vi "Untitled 1.vi"() -> ()   [LabVIEW 2018]
uses:
  <vilib>/userdefined/High Color/IMAQdx.ctl
  <vilib>/vision/driver/NI_Vision_Acquisition_Software.lvlib
  <resource>/objmgr/imaqdx.rc
  <vilib>/vision/NI_Vision_Development_Module.lvlib
panel:
  in  "Blue or Luma or Val or Inten Range":cluster{"Lower value":i32, "Upper value":i32}={"Lower value"=0, "Upper value"=255}
  in  "Green or Sat Range":cluster{"Lower value":i32, "Upper value":i32}={"Lower value"=0, "Upper value"=255}
  in  "Red or Hue Range":cluster{"Lower value":i32, "Upper value":i32}={"Lower value"=0, "Upper value"=255}
  in  "Stop (F)":bool
  out "Image Out":T1(plugin-control)
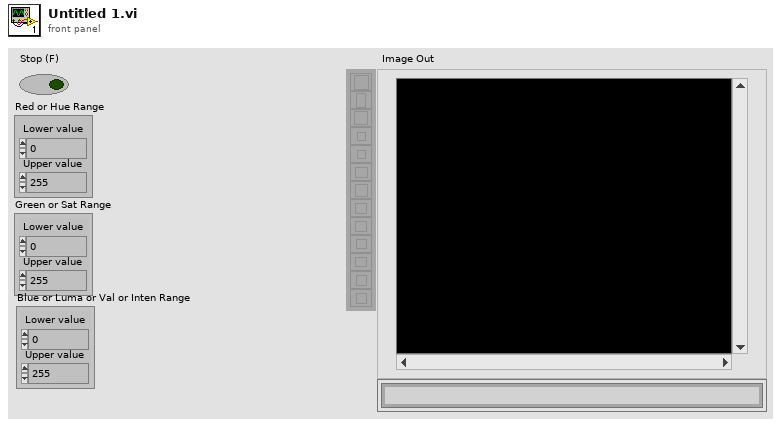
[diagram p1: front panel]
types:
  T1 = typedef "IMAQ Image.ctl" = refnum<image>
  T2 = typedef "IMAQdx.ctl" = refnum<k21>
  T3 = typedef "Particle Parameters" = i32
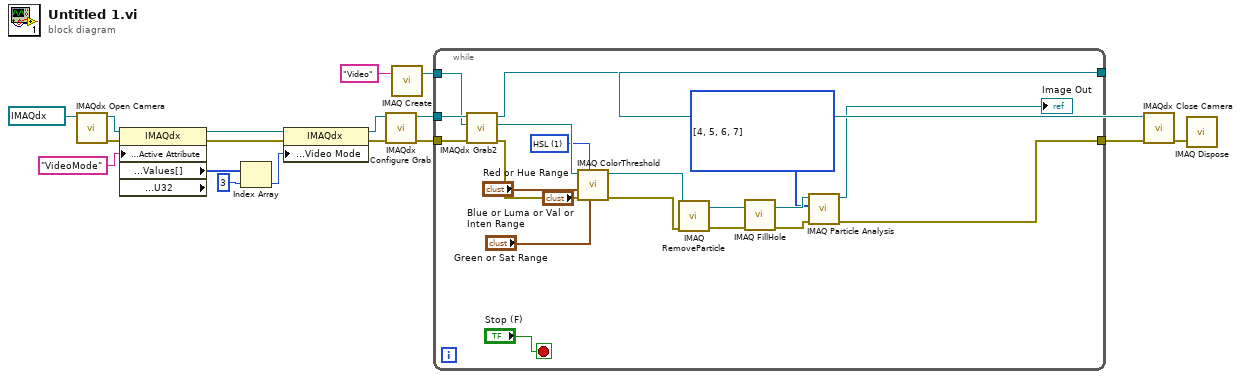
[diagram p0: block diagram]
diagram:
  n1 = call <vilib>:"IMAQdx Open Camera.vi"("Session In"=T2 "cam4") -> ("error out"=w4:errorcluster, "Session Out"=w5:T2)  [unwired: 9 in]
  n2 = property class="IMAQdx" props=["Camera Attributes:Active Attribute", "Camera Attributes:Enum:Values[]", "Camera Attributes:Value:U32"](reference=w5, error in=w4, "Camera Attributes:Active Attribute"="VideoMode" ("ActiveAttribute")) -> (reference out=w7:T2, error out=w8:errorcluster, "Camera Attributes:Enum:Values[]"=w11:u32[])  [unwired: 1 out]
  n3 = Index Array(array=w11, index=3 ("Video Modes")) -> (element=w10:u32)
  n4 = property class="IMAQdx"(reference=w7, error in=w8, "Acquisition Attributes:Video Mode"=w10) -> (reference out=w3:T2, error out=w2:errorcluster)
  n5 = call <vilib>:"IMAQdx Configure Grab.vi"("error in"=w2, "Session In"=w3) -> ("error out"=w17:errorcluster, "Session Out"=w16:T2)  [unwired: 8 in]
  n6 = call "IMAQ Create"("Image Name"="Video") -> ("New Image"=w14:T1)  [unwired: 4 in, 1 out]
  n7 = while {
    tunnel: [w37] -> w18
    tunnel: w17 -> [w36]
    tunnel: w16 -> [w35]
    tunnel: w14 -> [w34]
    tunnel: [w19] -> w1
    stop <- "Stop (F)" stop-if-true
    w21 = T3[] [4, 5, 6, 7] items=["Center of Mass X", "Center of Mass Y", "First Pixel X", "First Pixel Y", "Bounding Rect Left", "Bounding Rect Top", "Bounding Rect Right", "Bounding Rect Bottom", "Max Feret Diameter Start X", "Max Feret Diameter Start Y", "Max Feret Diameter End X", "Max Feret Diameter End Y", "Max Horiz. Segment Length Left", "Max Horiz. Segment Length Right", "Max Horiz. Segment Length Row", "-", "Bounding Rect Width", "Bounding Rect Height", "Bounding Rect Diagonal", "Perimeter", "Convex Hull Perimeter", "Holes' Perimeter", "Max Feret Diameter", "Equivalent Ellipse Major Axis", "Equivalent Ellipse Minor Axis", "Equivalent Ellipse Minor Axis (Feret)", "Equivalent Rect Long Side", "Equivalent Rect Short Side", "Equivalent Rect Diagonal", "Equivalent Rect Short Side (Feret)", "Average Horiz. Segment Length", "Average Vert. Segment Length", "Hydraulic Radius", "Waddel Disk Diameter", "-", "Area", "Holes' Area", "Particle & Holes' Area", "Convex Hull Area", "Image Area", "-", "Number of Holes", "Number of Horiz. Segments", "Number of Vert. Segments", "-", "Orientation", "Max Feret Diameter Orientation", "-", "% Area/Image Area", "% Area/(Particle & Holes' Area)", "Ratio of Equivalent Ellipse Axes", "Ratio of Equivalent Rect Sides", "-", "Elongation Factor", "Compactness Factor", "Heywood Circularity Factor", "Type Factor", "-", "Sum X", "Sum Y", "Sum XX", "Sum XY", "Sum YY", "Sum XXX", "Sum XXY", "Sum XYY", "Sum YYY", "-", "Moment of Inertia XX", "Moment of Inertia XY", "Moment of Inertia YY", "Moment of Inertia XXX", "Moment of Inertia XXY", "Moment of Inertia XYY", "Moment of Inertia YYY", "Norm. Moment of Inertia XX", "Norm. Moment of Inertia XY", "Norm. Moment of Inertia YY", "Norm. Moment of Inertia XXX", "Norm. Moment of Inertia XXY", "Norm. Moment of Inertia XYY", "Norm. Moment of Inertia YYY", "Hu Moment 1", "Hu Moment 2", "Hu Moment 3", "Hu Moment 4", "Hu Moment 5", "Hu Moment 6", "Hu Moment 7"] ("Pixel Measurements")
    w31 = u16 1 items=["RGB", "HSL", "HSV", "HSI"] ("Color Mode")
    n8 = call <vilib>:"IMAQdx Grab2.vi"("error in"=w36, "Image In"=w34, "Session In"=w35) -> ("error out"=w33:errorcluster, "Image Out"=w32:T1, "Session Out"=w37:T2)  [unwired: 5 in, 1 out]
    n9 = call "IMAQ ColorThreshold"("Blue or Luma or Val or Inten Range"="Blue or Luma or Val or Inten Range", "Green or Sat Range"="Green or Sat Range", "Color Mode"=w31, "error in (no error)"=w33, "Red or Hue Range"="Red or Hue Range", "Image Src"=w32) -> ("error out"=w27:errorcluster, "Image Dst Out"=w26:T1)  [unwired: 4 in]
    n10 = call "IMAQ RemoveParticle"("error in (no error)"=w27, "Image Src"=w26) -> ("error out"=w24:errorcluster, "Image Dst Out"=w25:T1)  [unwired: 8 in]
    n11 = call "IMAQ FillHole"("error in (no error)"=w24, "Image Src"=w25) -> ("error out"=w22:errorcluster, "Image Dst Out"=w23:T1)  [unwired: 4 in]
    n12 = call "IMAQ Particle Analysis"("error in (no error)"=w22, "Pixel Measurements"=w21, "Image"=w23) -> ("error out"=w19:errorcluster, "Image Out (duplicate)"=→"Image Out":T1)  [unwired: 3 in, 4 out]
  }
  n13 = call <vilib>:"IMAQdx Close Camera.vi"("error in"=w1, "Session In"=w18) -> ("error out"=w13:errorcluster)  [unwired: 9 in]
  n14 = call "IMAQ Dispose"("error in (no error)"=w13) -> ()  [unwired: 5 in, 1 out]
